vi "ZBX Antenna to Register Offset.vi"(11 "Antenna":T1) -> (3 "register offset":u32)   [LabVIEW 2023]
uses:
  <instrlib>/niUSRP/Reference FPGA/ZBX Control/Antenna.ctl
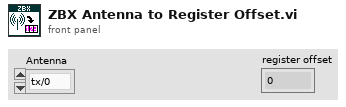
[diagram p1: front panel]
types:
  T1 = typedef "Antenna.ctl" = enum8{"tx/0", "tx/1", "rx/0", "rx/1"}
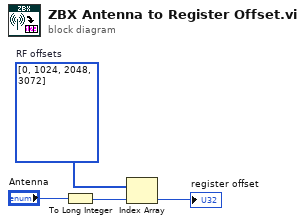
[diagram p0: block diagram]
diagram:
  w3 = u32[] [0, 1024, 2048, 3072]  # RF offsets
  n1 = To Long Integer(number="Antenna") -> (32bit integer=w2:i32)
  n2 = Index Array(array=w3, index=w2) -> (element=→"register offset":u32)
